vi "simuate LIDAR.vi"() -> ()   [LabVIEW 2009]
uses:
  <vilib>/Utility/miscctls.llb/LVPoint32TypeDef.ctl
panel:
  in  "stop":bool
  in  "Tab Control":enum32{"setup", "picture", "graph"}(tab)
  in  "Cluster":T1={"color diff"=TRUE, "foreground"=1191935, "background"=14455040}
  out "error out":errorcluster
  in  "update":bool
  in  "Image path":path
  in  "sample resolution":i32=100
  out "2D Picture":picture
  out "Coords":T2
  out "Waveform Graph":sgl[](graph)
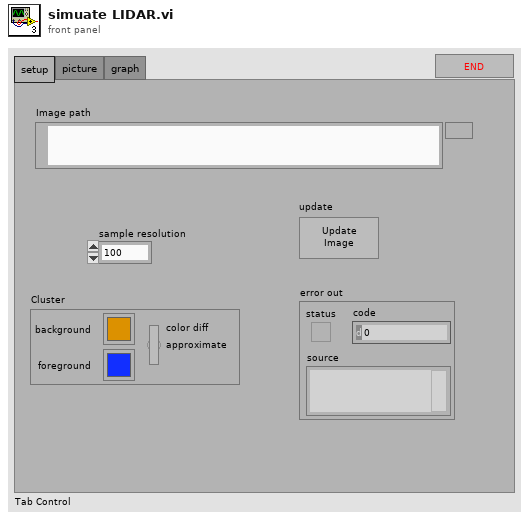
[diagram p1: front panel]
types:
  T1 = cluster{"color diff":bool, "foreground":u32, "background":u32}
  T2 = typedef "LVPoint32TypeDef.ctl" = cluster{"Horizontal":i32, "Vertical":i32}
  T3 = typedef "LVPositionTypeDef.ctl" = cluster{"Left":i32, "Top":i32}
  T4 = typedef "LVPointTypeDef.ctl" = cluster{"Horizontal":i16, "Vertical":i16}
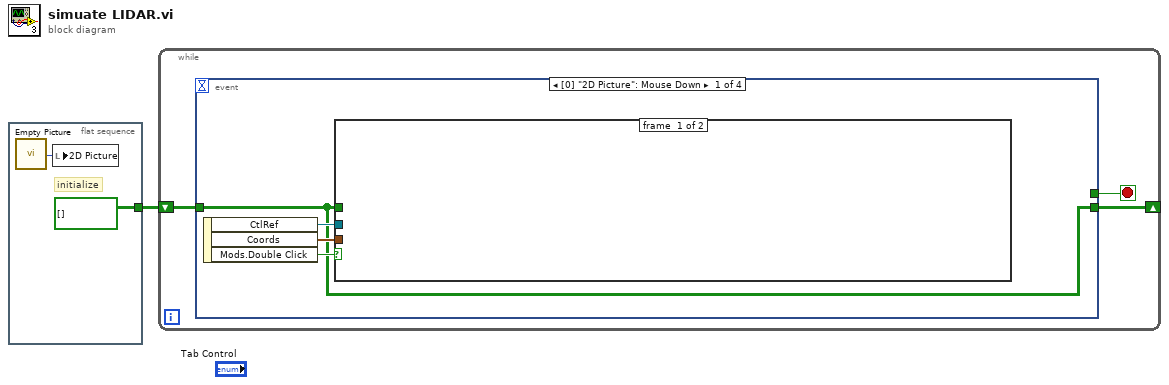
[diagram p0: block diagram]
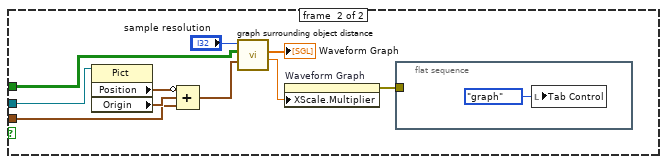
[diagram p2: hidden frame]
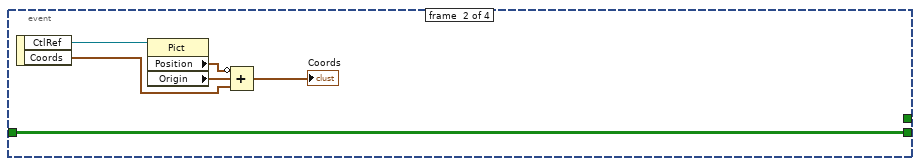
[diagram p3: hidden frame]
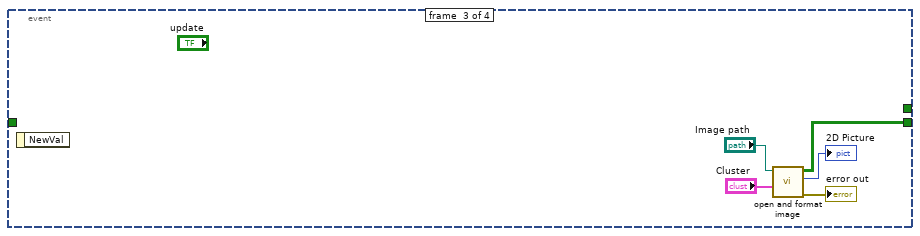
[diagram p4: hidden frame]
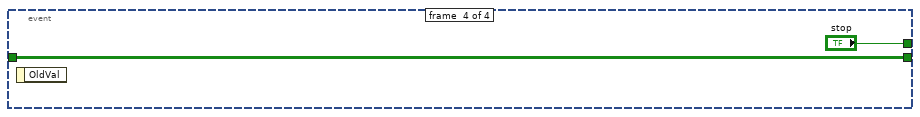
[diagram p5: hidden frame]
diagram:
  n1 = flat-sequence {
    tunnel: [bool[][] [] ("1-bit pixmap")] -> w1
    frame #0 {
      # "initialize"
      n2 = call "Empty Picture"() -> ("empty picture"=w3:picture)
      n3 = local write "2D Picture"(w3) -> ()
    }
  }
  n4 = while {
    shift-right: [w5] -> _
    shift-left: w1 -> [w4]
    stop <- w6 stop-if-true
    n5 = event shown="[0] \"2D Picture\": Mouse Down" {
      selector: _ -> [_ _ _ _]
      dyn-events: _ -> [_ _ _ _]
      timeout: _ -> [_ _ _ _]
      tunnel: [_ _ _ "stop"] -> w6
      tunnel: [w7 w22 w28 w33] -> w5
      tunnel: w4 -> [w7 w22 _ w33]
      event #0 {
        n6 = event-data() -> ("CtlRef"=w10:refnum<vi>, "Coords"=w9:T2, "Mods.Double Click"=w8:bool)  [unwired: 1 in]
        n7 = case shown="True" w8 {
          tunnel: w10 -> [_ w20]
          tunnel: w9 -> [_ w17]
          tunnel: w7 -> [_ w12]
          frame #0 {
          }
          frame #1 {
            n8 = property class="Pict"(reference=w20) -> ("Position"=w18:T3, "Origin"=w19:T4)  [unwired: 1 in, 2 out]
            n9 = Compound Arithmetic op=ADD(invert w18, w19, w17) -> (w16:T3)
            n10 = call "graph surrounding object distance.vi"("point"=w16, "raster image"=w12, "sample resolution"="sample resolution") -> ("scale multiplier"=w14:dbl, "Waveform Graph"=→"Waveform Graph":sgl[])  [unwired: 7 in]
            n11 = property on="Waveform Graph" class="WFGraph (strict)"("XScale.Multiplier"=w14) -> (error out=w11:errorcluster)  [unwired: 2 in, 1 out]
            n12 = flat-sequence {
              tunnel: w11 -> [_]
              frame #0 {
                n13 = local write "Tab Control"(enum32{"setup", "picture", "graph"}."graph" ("Tab Control")) -> ()
              }
            }
          }
        }
      }
      event #1 {
        n14 = event-data() -> ("CtlRef"=w25:refnum<vi>, "Coords"=w24:T2)  [unwired: 1 in]
        n15 = property class="Pict"(reference=w25) -> ("Position"=w26:T3, "Origin"=w27:T4)  [unwired: 1 in, 2 out]
        n16 = Compound Arithmetic op=ADD(invert w26, w27, w24) -> (→"Coords":T3)
      }
      event #2 {
        n17 = event-data() -> ()  [unwired: 1 in, 1 out]
        n18 = call "open and format image.vi"("colors"="Cluster", "Image path"="Image path") -> ("error out"=→"error out":errorcluster, "2D Picture"=→"2D Picture":picture, "1-bit pixmap"=w28:bool[][])  [unwired: 7 in]
      }
      event #3 {
        n19 = event-data() -> ()  [unwired: 1 in, 1 out]
      }
    }
  }
